vi "M686_Quit.vi"(11 "VISA Refnum in":refnum<visa-resource-name>) -> ()   [LabVIEW 2014]
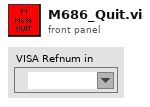
[diagram p1: front panel]
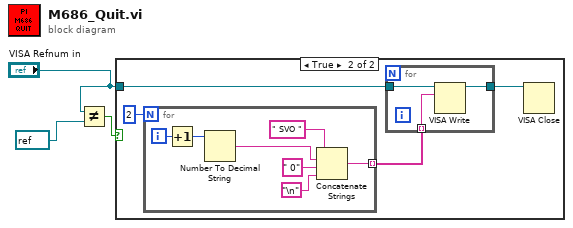
[diagram p0: block diagram]
diagram:
  n1 = Not Equal?(x="VISA Refnum in", y=refnum<visa-resource-name> refnum ("VISA resource name")) -> (x != y?=w1:bool)
  n2 = case shown="True" w1 {
    tunnel: "VISA Refnum in" -> [_ w7]
    frame False {
    }
    frame True {
      n3 = for {
        N: 2 -> [_]
        tunnel: [w17] -> w4 mode=indexing
        i -> [w14]
        n4 = Increment(x=w14) -> (x+1=w15:i32)
        n5 = Number To Decimal String(number=w15) -> (decimal integer string=w11:string)  [unwired: 1 in]
        n6 = Concatenate Strings(" SVO " ("string"), w11, " 0" ("string"), "\n") -> (w17:string)
      }
      n7 = for {
        tunnel: w7 -> [w10]
        tunnel: [w9] -> w5
        tunnel: w4 -> [w8] mode=indexing
        n8 = VISA Write(VISA resource name=w10, write buffer=w8) -> (VISA resource name out=w9:refnum<visa-resource-name>)  [unwired: 1 in, 2 out]
      }
      n9 = VISA Close(VISA resource name=w5) -> ()  [unwired: 1 in, 1 out]
    }
  }
